vi "Launch Message Handler.vi"(8 "error in (no error)":errorcluster, 10 "stop notifier":refnum<notifier>, 11 "message queue in":refnum<queue>) -> (0 "error out":errorcluster)   [LabVIEW 2020, in "Frame Logging.lvlib"]
uses:
  Frame Logging.lvlib
  Message_Request.ctl
  Message_Request_Action.ctl
  Message Handler.vi
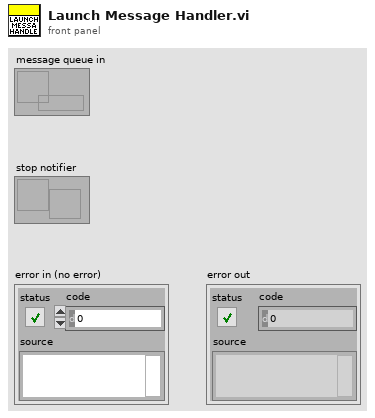
[diagram p1: front panel]
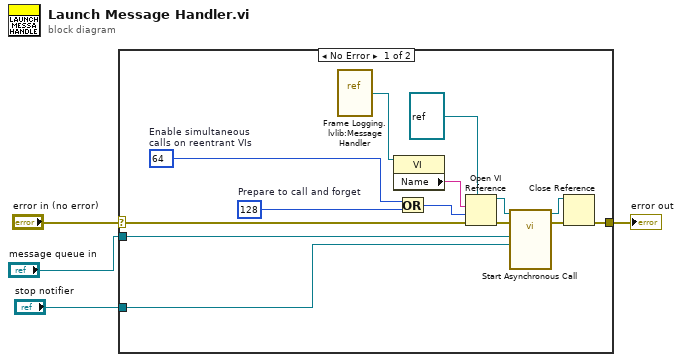
[diagram p0: block diagram]
diagram:
  n1 = case shown="No Error" "error in (no error)" {
    selector: "error in (no error)" -> [w18 w19]
    tunnel: [w8 w19] -> w3
    tunnel: "message queue in" -> [w6 _]
    tunnel: "stop notifier" -> [w5 _]
    frame No Error {
      w13 = 64  # Enable simultaneous calls on reentrant VIs
      w14 = 128  # Prepare to call and forget
      n2 = vi-ref "Frame Logging.lvlib:Message Handler.vi"() -> (w11:refnum<vi>)
      n3 = property class="VI"(reference=w11) -> ("Name"=w9:string)  [unwired: 1 in, 2 out]
      n4 = Or(x=w13, y=w14) -> (x .or. y?=w12:i32)
      n5 = Open VI Reference(type specifier VI Refnum (for type only)=refnum<vi> refnum, vi path=w9, options=w12, error in (no error)=w18) -> (vi reference=w17:refnum<vi>, error out=w16:errorcluster)  [unwired: 2 in]
      n6 = call-by-ref "Start Asynchronous Call"(reference=w17, error in=w16, "stop notifier"=w5, "Messages in"=w6) -> (reference out=w7:refnum<vi>, error out=w15:errorcluster)  [unwired: 10 in]
      n7 = Close Reference(reference=w7, error in (no error)=w15) -> (error out=w8:errorcluster)
    }
    frame Error {
    }
  }
  "error out" <- w3
